vi "test RT to RT with Start Stop and Status.vi"(8 "error in":errorcluster, 11 "Loopback in":refnum<class "Loopback.lvclass">) -> (0 "error out":errorcluster, 3 "Loopback out":refnum<class "Loopback.lvclass">)   [LabVIEW 2020, in "Loopback.lvclass"]
uses:
  Loopback.lvclass
  C:/Program Files (x86)/National Instruments/LabVIEW 2020/vi.lib/NI/VeriStand Custom Device Testing Tools/VeriStandTestCase/VeriStandTestCase.lvclass
  <vilib>/numeric/Random Number (Range) U64.vi
  f971646f-b932-43f4-9b5e-09c05c27b744.vi
  c977f9e6-6c4f-4805-a1b3-4d712966c110.vi
  51cd3b25-3203-4dc5-9c8f-cd86cb6b692f.vi
  <vilib>/numeric/sub_Random U32.vi
  <vilib>/NI VeriStand/Execution/Workspace/NI VeriStand - Get Multiple Channel Values.vi
  <vilib>/NI VeriStand/Execution/Workspace/NI VeriStand - Set Single Channel Value.vi
  <vilib>/NI VeriStand/Execution/Workspace/NI VeriStand - Get Single Channel Value.vi
  <vilib>/NI VeriStand/Execution/Workspace/NI VeriStand - Set Multiple Channel Values.vi
  <vilib>/NI VeriStand/Execution/Workspace/NI_VS Workspace ExecutionAPI.lvlib
  <vilib>/NI/VeriStand Custom Device Testing Tools/VeriStandTestUtilities/VeriStandTestUtilities.lvlib
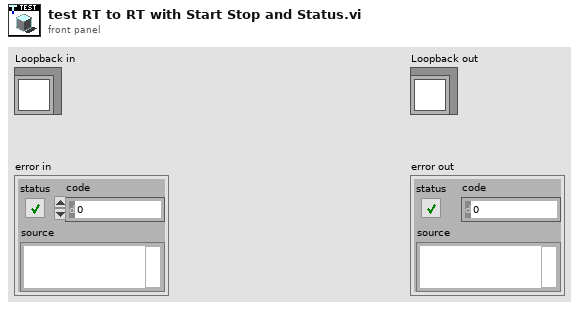
[diagram p1: front panel]
types:
  T1 = typedef "NI_VS Workspace ExecutionAPI.lvlib/WorkspaceAPI.ctl" = refnum<k24>
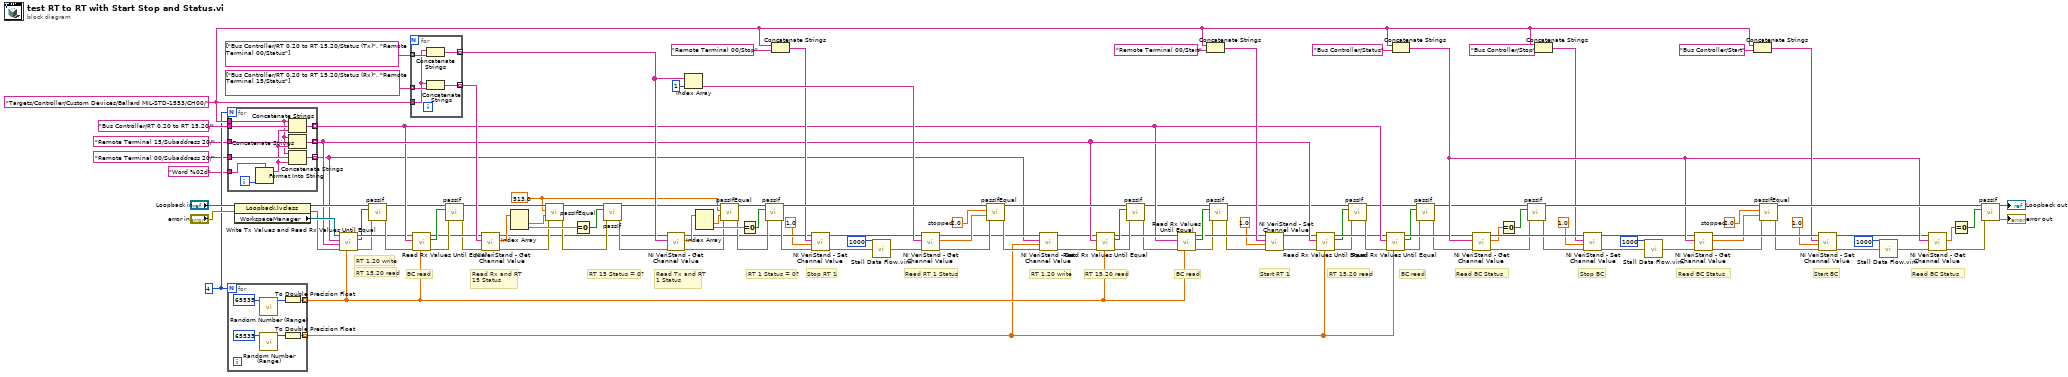
[diagram p0: block diagram]
diagram:
  w112 = "Targets/Controller/Custom Devices/Ballard MIL-STD-1553/CH00/" ("base name for channel aliases")
  w88 = 2.0  # stopped
  w84 = 2.0  # stopped
  w3 = 513.0 ("element")
  w11 = 4
  # "Start BC"
  # "Read BC Status"
  # "Stop BC"
  # "Read BC Status"
  # "Read BC Status"
  # "Read RT 1 Status"
  # "RT 1 Status = 0?"
  # "RT 15 Status = 0?"
  # "Read Tx and RT 1 Status"
  # "Read Rx and RT 15 Status"
  # "BC read"
  # "RT 15.20 read"
  # "BC read"
  # "RT 15.20 read"
  # "RT 1.20 write"
  # "BC read"
  # "RT 15.20 read"
  # "RT 1.20 write"
  # "Start RT 1"
  # "Stop RT 1"
  n1 = for {
    N: w11 -> [_]
    tunnel: "Remote Terminal 00/Subaddress 20/" ("Channel") -> [w135]
    tunnel: [w136] -> w26 mode=indexing
    tunnel: "Remote Terminal 15/Subaddress 20/" ("Channel") -> [w134]
    tunnel: [w133] -> w50 mode=indexing
    tunnel: "Word %02d" -> [w128]
    tunnel: "Bus Controller/RT 0.20 to RT 15.20/" ("Channel") -> [w131]
    tunnel: [w129] -> w43 mode=indexing
    tunnel: w112 -> [w127]
    i -> [w132]
    n2 = Format Into String(format string=w128, w132) -> (resulting string=w130:string)  [unwired: 2 in, 1 out]
    n3 = Concatenate Strings(w127, w131, w130) -> (w129:string)
    n4 = Concatenate Strings(w127, w134, w130) -> (w133:string)
    n5 = Concatenate Strings(w127, w135, w130) -> (w136:string)
  }
  n6 = for {
    N: w11 -> [_]
    tunnel: [w140] -> w41 mode=indexing
    tunnel: [w137] -> w54 mode=indexing
    n7 = call-poly <vilib>:"Random Number (Range).vi"("upper bound (100)"=u64 65535) -> ("number"=w139:u64)  [unwired: 10 in]
    n8 = call-poly <vilib>:"Random Number (Range).vi"("upper bound (100)"=u64 65535) -> ("number"=w141:u64)  [unwired: 10 in]
    n9 = To Double Precision Float(number=w139) -> (double precision float=w137:dbl)
    n10 = To Double Precision Float(number=w141) -> (double precision float=w140:dbl)
  }
  n11 = property class="Loopback.lvclass"(reference="Loopback in", error in="error in") -> (reference out=w125:refnum<class "Loopback.lvclass">, error out=w123:errorcluster, "WorkspaceManager"=w126:T1)
  n12 = call <vilib>:"Write Tx Values and Read Rx Values Until Equal.vi"("Tx values"=w54, "error in"=w123, "Rx aliases"=w50, "Tx aliases"=w26, "workspace manager in"=w126) -> ("error out"=w27:errorcluster, "values equal"=w28:bool, "workspace manager out"=w29:T1)  [unwired: 4 in]
  n13 = call-dynamic "passIf.vi"("error in (no error)"=w27, "pass"=w28, "TestCase in"=w125) -> ("error out"=w30:errorcluster, "TestCase out"=w13:refnum<class "Loopback.lvclass">)  [unwired: 7 in]
  n14 = for {
    tunnel: [w147] -> w57 mode=indexing
    tunnel: [w146] -> w76 mode=indexing
    tunnel: string[] ["Bus Controller/RT 0.20 to RT 15.20/Status (Tx)", "Remote Terminal 00/Status"] -> [w145] mode=indexing
    tunnel: string[] ["Bus Controller/RT 0.20 to RT 15.20/Status (Rx)", "Remote Terminal 15/Status"] -> [w144] mode=indexing
    tunnel: w112 -> [w143]
    n15 = Concatenate Strings(w143, w145) -> (w146:string)
    n16 = Concatenate Strings(w143, w144) -> (w147:string)
  }
  n17 = call <vilib>:"Read Rx Values Until Equal.vi"("expected values"=w54, "error in"=w30, "Rx aliases"=w43, "workspace manager in"=w29) -> ("error out"=w32:errorcluster, "values equal expected"=w33:bool, "workspace manager out"=w31:T1)  [unwired: 5 in]
  n18 = call-dynamic "passIf.vi"("error in (no error)"=w32, "pass"=w33, "TestCase in"=w13) -> ("error out"=w21:errorcluster, "TestCase out"=w22:refnum<class "Loopback.lvclass">)  [unwired: 7 in]
  n19 = call-poly <vilib>:"NI VeriStand - Get Channel Value.vi"("error in (no error)"=w21, "Channels"=w57, "WorkspaceManager in"=w31) -> ("error out"=w20:errorcluster, "Values"=w25:dbl[], "WorkspaceManager out"=w18:T1)  [unwired: 6 in]
  n20 = Index Array(array=w25) -> (element #1=w1:dbl, element #2=w66:dbl)  [unwired: 2 in]
  n21 = call-dynamic "passIfEqual.vi"("error in (no error)"=w20, "y"=w1, "x"=w3, "TestCase in"=w22) -> ("error out"=w62:errorcluster, "TestCase out"=w64:refnum<class "Loopback.lvclass">)  [unwired: 6 in]
  n22 = Equal To 0?(x=w66) -> (x = 0?=w67:bool)
  n23 = call-dynamic "passIf.vi"("error in (no error)"=w62, "pass"=w67, "TestCase in"=w64) -> ("error out"=w63:errorcluster, "TestCase out"=w65:refnum<class "Loopback.lvclass">)  [unwired: 7 in]
  n24 = call-poly <vilib>:"NI VeriStand - Get Channel Value.vi"("error in (no error)"=w63, "Channels"=w76, "WorkspaceManager in"=w18) -> ("error out"=w19:errorcluster, "Values"=w24:dbl[], "WorkspaceManager out"=w23:T1)  [unwired: 6 in]
  n25 = Index Array(array=w76, index=1) -> (element=w78:string)
  n26 = Index Array(array=w24) -> (element #1=w2:dbl, element #2=w72:dbl)  [unwired: 2 in]
  n27 = call-dynamic "passIfEqual.vi"("error in (no error)"=w19, "y"=w2, "x"=w3, "TestCase in"=w65) -> ("error out"=w70:errorcluster, "TestCase out"=w69:refnum<class "Loopback.lvclass">)  [unwired: 6 in]
  n28 = Equal To 0?(x=w72) -> (x = 0?=w68:bool)
  n29 = call-dynamic "passIf.vi"("error in (no error)"=w70, "pass"=w68, "TestCase in"=w69) -> ("error out"=w71:errorcluster, "TestCase out"=w79:refnum<class "Loopback.lvclass">)  [unwired: 7 in]
  n30 = Concatenate Strings(w112, "Remote Terminal 00/Stop" ("Channel")) -> (w59:string)
  n31 = call-poly <vilib>:"NI VeriStand - Set Channel Value.vi"("error in (no error)"=w71, "Value"=1.0, "Channel"=w59, "WorkspaceManager in"=w23) -> ("error out"=w10:errorcluster, "WorkspaceManager out"=w73:T1)  [unwired: 6 in]
  n32 = call "Stall Data Flow.vim"("value in"=w10, "milliseconds to wait"=u32 1000) -> ("value out"=w74:errorcluster)  [unwired: 1 out]
  n33 = call-poly <vilib>:"NI VeriStand - Get Channel Value.vi"("error in (no error)"=w74, "Channel"=w78, "WorkspaceManager in"=w73) -> ("error out"=w81:errorcluster, "Value"=w83:dbl, "WorkspaceManager out"=w75:T1)  [unwired: 6 in]
  n34 = call-dynamic "passIfEqual.vi"("error in (no error)"=w81, "y"=w83, "x"=w84, "TestCase in"=w79) -> ("error out"=w82:errorcluster, "TestCase out"=w80:refnum<class "Loopback.lvclass">)  [unwired: 6 in]
  n35 = call-poly <vilib>:"NI VeriStand - Set Channel Value.vi"("error in (no error)"=w82, "Values"=w41, "Channels"=w26, "WorkspaceManager in"=w75) -> ("error out"=w49:errorcluster, "WorkspaceManager out"=w48:T1)  [unwired: 6 in]
  n36 = call <vilib>:"Read Rx Values Until Equal.vi"("expected values"=w54, "error in"=w49, "Rx aliases"=w50, "workspace manager in"=w48) -> ("error out"=w52:errorcluster, "values equal expected"=w53:bool, "workspace manager out"=w51:T1)  [unwired: 5 in]
  n37 = call-dynamic "passIf.vi"("error in (no error)"=w52, "pass"=w53, "TestCase in"=w80) -> ("error out"=w44:errorcluster, "TestCase out"=w16:refnum<class "Loopback.lvclass">)  [unwired: 7 in]
  n38 = call <vilib>:"Read Rx Values Until Equal.vi"("expected values"=w54, "error in"=w44, "Rx aliases"=w43, "workspace manager in"=w51) -> ("error out"=w45:errorcluster, "values equal expected"=w47:bool, "workspace manager out"=w46:T1)  [unwired: 5 in]
  n39 = Concatenate Strings(w112, "Remote Terminal 00/Start" ("Channel")) -> (w61:string)
  n40 = call-dynamic "passIf.vi"("error in (no error)"=w45, "pass"=w47, "TestCase in"=w16) -> ("error out"=w15:errorcluster, "TestCase out"=w17:refnum<class "Loopback.lvclass">)  [unwired: 7 in]
  n41 = call-poly <vilib>:"NI VeriStand - Set Channel Value.vi"("error in (no error)"=w15, "Value"=1.0, "Channel"=w61, "WorkspaceManager in"=w46) -> ("error out"=w35:errorcluster, "WorkspaceManager out"=w34:T1)  [unwired: 6 in]
  n42 = call <vilib>:"Read Rx Values Until Equal.vi"("expected values"=w41, "error in"=w35, "Rx aliases"=w50, "workspace manager in"=w34) -> ("error out"=w37:errorcluster, "values equal expected"=w36:bool, "workspace manager out"=w38:T1)  [unwired: 5 in]
  n43 = call-dynamic "passIf.vi"("error in (no error)"=w37, "pass"=w36, "TestCase in"=w17) -> ("error out"=w39:errorcluster, "TestCase out"=w14:refnum<class "Loopback.lvclass">)  [unwired: 7 in]
  n44 = call <vilib>:"Read Rx Values Until Equal.vi"("expected values"=w41, "error in"=w39, "Rx aliases"=w43, "workspace manager in"=w38) -> ("error out"=w40:errorcluster, "values equal expected"=w42:bool, "workspace manager out"=w93:T1)  [unwired: 5 in]
  n45 = Concatenate Strings(w112, "Bus Controller/Status" ("Channel")) -> (w110:string)
  n46 = call-dynamic "passIf.vi"("error in (no error)"=w40, "pass"=w42, "TestCase in"=w14) -> ("error out"=w92:errorcluster, "TestCase out"=w89:refnum<class "Loopback.lvclass">)  [unwired: 7 in]
  n47 = call-poly <vilib>:"NI VeriStand - Get Channel Value.vi"("error in (no error)"=w92, "Channel"=w110, "WorkspaceManager in"=w93) -> ("error out"=w91:errorcluster, "Value"=w90:dbl, "WorkspaceManager out"=w101:T1)  [unwired: 6 in]
  n48 = Equal To 0?(x=w90) -> (x = 0?=w85:bool)
  n49 = call-dynamic "passIf.vi"("error in (no error)"=w91, "pass"=w85, "TestCase in"=w89) -> ("error out"=w98:errorcluster, "TestCase out"=w120:refnum<class "Loopback.lvclass">)  [unwired: 7 in]
  n50 = Concatenate Strings(w112, "Bus Controller/Stop" ("Channel")) -> (w100:string)
  n51 = call-poly <vilib>:"NI VeriStand - Set Channel Value.vi"("error in (no error)"=w98, "Value"=1.0, "Channel"=w100, "WorkspaceManager in"=w101) -> ("error out"=w95:errorcluster, "WorkspaceManager out"=w102:T1)  [unwired: 6 in]
  n52 = call "Stall Data Flow.vim"("value in"=w95, "milliseconds to wait"=u32 1000) -> ("value out"=w103:errorcluster)  [unwired: 1 out]
  n53 = call-poly <vilib>:"NI VeriStand - Get Channel Value.vi"("error in (no error)"=w103, "Channel"=w110, "WorkspaceManager in"=w102) -> ("error out"=w86:errorcluster, "Value"=w87:dbl, "WorkspaceManager out"=w119:T1)  [unwired: 6 in]
  n54 = Concatenate Strings(w112, "Bus Controller/Start" ("Channel")) -> (w113:string)
  n55 = call-dynamic "passIfEqual.vi"("error in (no error)"=w86, "y"=w87, "x"=w88, "TestCase in"=w120) -> ("error out"=w109:errorcluster, "TestCase out"=w118:refnum<class "Loopback.lvclass">)  [unwired: 6 in]
  n56 = call-poly <vilib>:"NI VeriStand - Set Channel Value.vi"("error in (no error)"=w109, "Value"=1.0, "Channel"=w113, "WorkspaceManager in"=w119) -> ("error out"=w108:errorcluster, "WorkspaceManager out"=w105:T1)  [unwired: 6 in]
  n57 = call "Stall Data Flow.vim"("value in"=w108, "milliseconds to wait"=u32 1000) -> ("value out"=w104:errorcluster)  [unwired: 1 out]
  n58 = call-poly <vilib>:"NI VeriStand - Get Channel Value.vi"("error in (no error)"=w104, "Channel"=w110, "WorkspaceManager in"=w105) -> ("error out"=w115:errorcluster, "Value"=w121:dbl)  [unwired: 6 in, 1 out]
  n59 = Equal To 0?(x=w121) -> (x = 0?=w114:bool)
  n60 = call-dynamic "passIf.vi"("error in (no error)"=w115, "pass"=w114, "TestCase in"=w118) -> ("error out"=→"error out":errorcluster, "TestCase out"=→"Loopback out":refnum<class "Loopback.lvclass">)  [unwired: 7 in]
